vi "CallInputList.vi"(5 "list":string, 9 "Function in":refnum<class "GrowableFunction.lvclass">) -> (3 "Function out":refnum<class "GrowableFunction.lvclass">, 4 "call inputs":string[](array[string]))   [LabVIEW 2014, in "GrowableFunction.lvclass"]
uses:
  GrowableFunction.lvclass
  Python/Parsing/Python Functions.lvlib
  Terminal/Terminal.lvclass
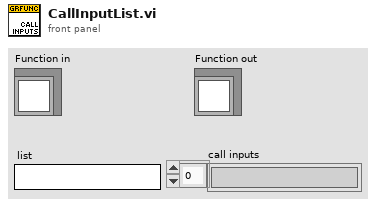
[diagram p1: front panel]
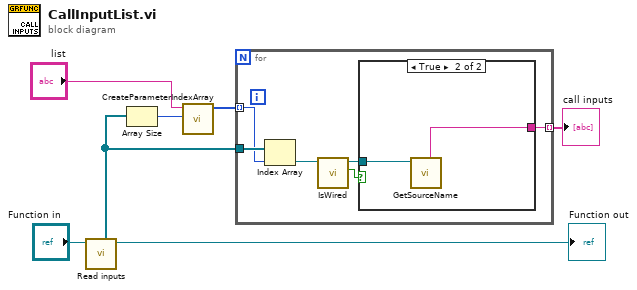
[diagram p0: block diagram]
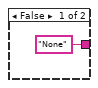
[diagram p2: hidden frame]
diagram:
  n1 = call-dynamic "Read inputs.vi"("Node in"="Function in") -> ("Node out"=→"Function out":refnum<class "GrowableFunction.lvclass">, "inputs"=w3:refnum<class "Terminal.lvclass">[])  [unwired: 7 in]
  n2 = Array Size(array=w3) -> (size(s)=w7:i32)
  n3 = call "CreateParameterIndexArray.vi"("length"=w7, "list"="list") -> ("Array"=w6:i32[])  [unwired: 9 in]
  n4 = for {
    tunnel: w6 -> [w12] mode=indexing
    tunnel: w3 -> [w13]
    tunnel: [w11] -> w1 mode=indexing
    n5 = Index Array(array=w13, index=w12) -> (element=w10:refnum<class "Terminal.lvclass">)
    n6 = call "IsWired.vi"("Terminal in"=w10) -> ("wired"=w8:bool, "Terminal out"=w9:refnum<class "Terminal.lvclass">)  [unwired: 6 in, 1 out]
    n7 = case shown="True" w8 {
      tunnel: ["None" w15] -> w11
      tunnel: w9 -> [_ w16]
      frame False {
      }
      frame True {
        n8 = call "GetSourceName.vi"("Terminal in"=w16) -> ("source"=w15:string)  [unwired: 6 in, 2 out]
      }
    }
  }
  "call inputs" <- w1
